vi "get Current Step.vi"(11 "Sequencer in":refnum<class "Sequencer.lvclass">) -> (3 "Current Step":string)   [LabVIEW 2020, in "Sequencer.lvclass"]
uses:
  Sequencer.lvclass
  Sequencer.lvclass/Sequencer.ctl
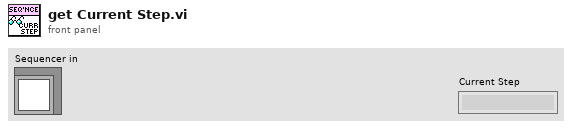
[diagram p1: front panel]
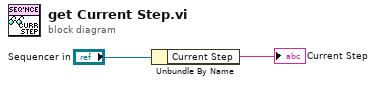
[diagram p0: block diagram]
diagram:
  n1 = Unbundle By Name("Sequencer in") -> ("Current Step"=→"Current Step":string)
